vi "GM Test Input Generator.vi"() -> ()   [LabVIEW 2010]
uses:
  <vilib>/DAQmx/write.llb/DAQmx Write (Analog DBL 1Chan 1Samp).vi
  <vilib>/DAQmx/create/channels.llb/DAQmx Create Channel (AO-Voltage-Basic).vi
  <vilib>/DAQmx/configure/timing.llb/DAQmx Timing (Sample Clock).vi
  <vilib>/daqmx/miscellaneous.llb/DAQmx Fill In Error Info.vi
panel:
  in  "Number of Steps":i32=500
  in  "Pulse Height (V)":dbl=-0.04
  in  "Count Rate (Hz)":u32=5 min=1
  in  "stop":bool
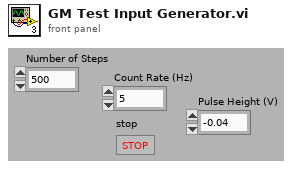
[diagram p1: front panel]
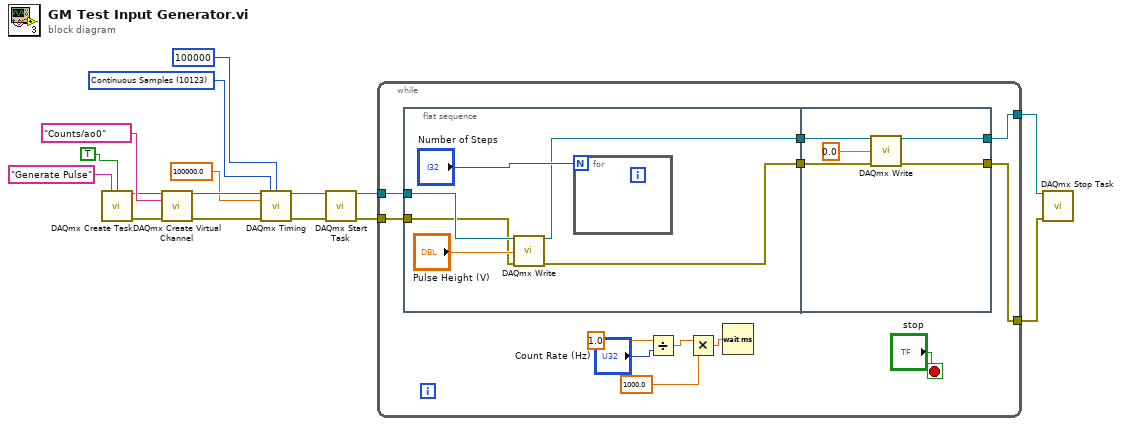
[diagram p0: block diagram]
diagram:
  w11 = 10123 items=["Finite Samples"=10178, "Continuous Samples"=10123, "Hardware Timed Single Point"=12522] ("sample mode")
  n1 = call <vilib>:"DAQmx Create Task.vi"("new task name"="Generate Pulse", "auto cleanup"=TRUE) -> ("task out"=w13:refnum<k21>, "error out"=w12:errorcluster)  [unwired: 12 in]
  n2 = call-poly <vilib>:"DAQmx Create Virtual Channel.vi"("task in"=w13, "physical channels"=tag "Counts/ao0", "error in"=w12) -> ("task out"=w10:refnum<k21>, "error out"=w9:errorcluster)  [unwired: 11 in]
  n3 = call-poly <vilib>:"DAQmx Timing.vi"("task/channels in"=w10, "sample mode"=w11, "samples per channel"=100000, "rate"=100000.0 ("Sample Clock Rate (Hz)"), "error in"=w9) -> ("task out"=w8:refnum<k21>, "error out"=w6:errorcluster)  [unwired: 9 in]
  n4 = call <vilib>:"DAQmx Start Task.vi"("task/channels in"=w8, "error in"=w6) -> ("task out"=w7:refnum<k21>, "error out"=w5:errorcluster)  [unwired: 12 in]
  n5 = while {
    tunnel: w7 -> [w28]
    tunnel: w5 -> [w27]
    tunnel: [w22] -> w2
    tunnel: [w23] -> w1
    stop <- "stop" stop-if-true
    n6 = flat-sequence {
      tunnel: w28 -> [w32]
      tunnel: w27 -> [w31]
      tunnel: [w30] -> w25
      tunnel: [w29] -> w24
      tunnel: w25 -> [w39]
      tunnel: w24 -> [w38]
      tunnel: [w36] -> w23
      tunnel: [w35] -> w22
      frame #0 {
        n7 = call-poly <vilib>:"DAQmx Write.vi"("task/channels in"=w32, "data"="Pulse Height (V)", "error in"=w31) -> ("task out"=w30:refnum<k21>, "error out"=w29:errorcluster)  [unwired: 10 in, 1 out]
        n8 = for {
          N: "Number of Steps" -> [_]
        }
      }
      frame #1 {
        n9 = call-poly <vilib>:"DAQmx Write.vi"("task/channels in"=w39, "data"=0.0, "error in"=w38) -> ("task out"=w35:refnum<k21>, "error out"=w36:errorcluster)  [unwired: 10 in, 1 out]
      }
    }
    n10 = Divide(x=1.0, y="Count Rate (Hz)") -> (x/y=w20:dbl)
    n11 = Multiply(x=w20, y=1000.0) -> (x*y=w19:dbl)
    n12 = Wait (ms)(milliseconds to wait=w19) -> ()  [unwired: 1 out]
  }
  n13 = call <vilib>:"DAQmx Stop Task.vi"("task/channels in"=w2, "error in"=w1) -> ()  [unwired: 12 in, 2 out]
